vi "MHTTP_CS_Http_request.vi"(6 "timeout":i32=2000, 7 "Method":enum16{"Version", "GET", "POST"}(ring), 8 "Error In":errorcluster, 10 "Data":string, 11 "URL in":string) -> (0 "Error Out":errorcluster, 3 "Response":string)   [LabVIEW 2018]
uses:
  D:/GitHub/MOKO/SE/Data/HttpRequestHelper.dll
  SE/Data/HttpRequestHelper.dll
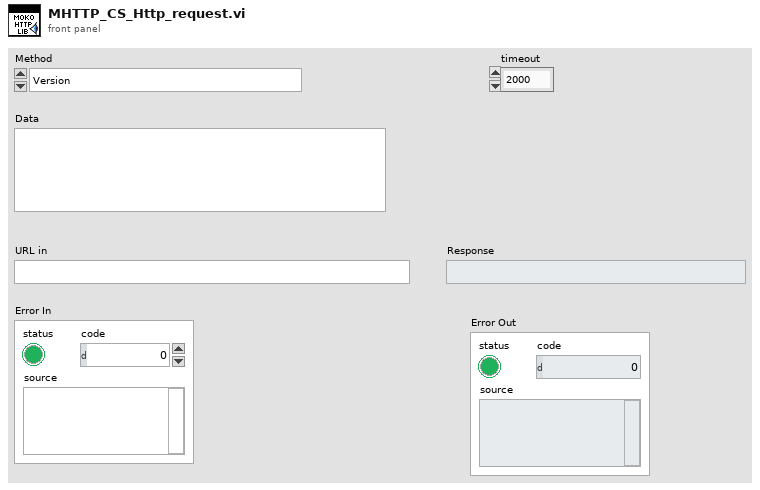
[diagram p1: front panel]
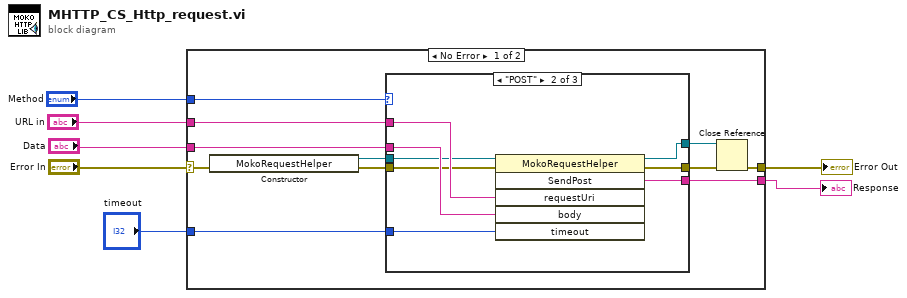
[diagram p0: block diagram]
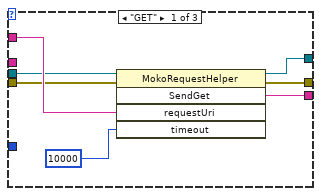
[diagram p2: hidden frame]
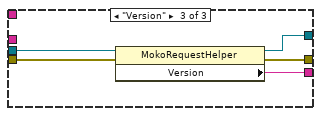
[diagram p3: hidden frame]
diagram:
  n1 = case shown="No Error" "Error In" {
    selector: "Error In" -> [w11 w39]
    tunnel: "URL in" -> [w18 _]
    tunnel: [w12 w39] -> w4
    tunnel: "Data" -> [w17 _]
    tunnel: [w16 _] -> w7
    tunnel: "Method" -> [w15 _]
    tunnel: "timeout" -> [w8 _]
    frame No Error {
      n2 = constructor class="MokoRequestHelper"(error in=w11) -> (reference out=w10:refnum<k24>, error out=w9:errorcluster)  [unwired: 2 in, 1 out]
      n3 = case shown="\"POST\"" w15 {
        tunnel: w18 -> [w23 w32 _]
        tunnel: w17 -> [_ w31 _]
        tunnel: [w24 w33 w38] -> w16
        tunnel: [w22 w27 w35] -> w14
        tunnel: [w21 w28 w34] -> w13
        tunnel: w10 -> [w20 w29 w37]
        tunnel: w9 -> [w19 w30 w36]
        tunnel: w8 -> [_ w26 _]
        frame "GET" {
          n4 = invoke class="MokoRequestHelper" method="SendGet"(reference=w20, error in=w19, "requestUri"=w23, "timeout"=10000) -> (reference out=w21:refnum<k24>, error out=w22:errorcluster, "SendGet"=w24:string)  [unwired: 1 in, 2 out]
        }
        frame "POST" {
          n5 = invoke class="MokoRequestHelper" method="SendPost"(reference=w29, error in=w30, "requestUri"=w32, "body"=w31, "timeout"=w26) -> (reference out=w28:refnum<k24>, error out=w27:errorcluster, "SendPost"=w33:string)  [unwired: 1 in, 3 out]
        }
        frame "Version" {
          n6 = property class="MokoRequestHelper"(reference=w37, error in=w36) -> (reference out=w34:refnum<k24>, error out=w35:errorcluster, "Version"=w38:string)
        }
      }
      n7 = Close Reference(reference=w13, error in (no error)=w14) -> (error out=w12:errorcluster)
    }
    frame Error {
    }
  }
  "Response" <- w7
  "Error Out" <- w4
